vi "check if tag name exists.vi"(10 "name to locate":string, 11 "shared memory module configuration in":refnum<class "shared memory configuration.lvclass">) -> (0 "tag config":T1, 1 "index":i32, 2 "found?":bool, 3 "shared memory module configuration out":refnum<class "shared memory configuration.lvclass">)   [LabVIEW 2013, in "shared memory configuration.lvclass"]
doc: "***TODO***\n\n<B>Input Parameters</B>\n\n<B>name to locate</B> ***TODO***name to locate\n\n<B>shared memory module configuration in</B> ***TODO***shared memory module configuration in\n\n<B>Output Parameters</B>\n\n<B>tag config</B> ***TODO***tag config\n\n<B> * name</B> ***TODO***tag config.name\n\n<B> * data type</B> ***TODO***tag config.data type***enum values: Double,Single,I64,I32,I16,I8,U64,U32,U16,U8,Boolean,String,Array of Double,Array of Single,Array of I64,Array of I32,Array of I16,Array of I8,Array of U64,Array of U32,Array of U16,Array of U8,Array of Boolean,Array of String\n\n<B> * channel</B> ***TODO***tag config.channel\n\n<B>index</B> ***TODO***index\n\n<B>found?</B> ***TODO***found?\n\n<B>shared memory module configuration out</B> ***TODO***shared memory module configuration out"
uses:
  shared memory configuration.lvclass
  <vilib>/NI/Tag Bus Module Framework/channel/TBM channel.lvclass
  Line.ctl
  <vilib>/NI/Tag Bus/tag/Data Type.ctl
  <vilib>/NI/Tag Bus/tag/tag descriptor.lvclass
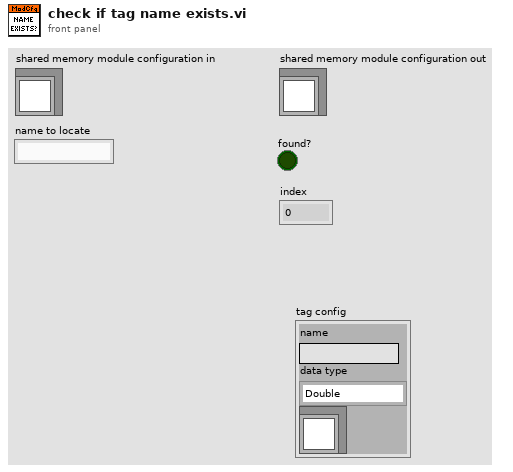
[diagram p1: front panel]
types:
  T1 = typedef "shared memory configuration.lvclass/Line.ctl" = cluster{"name":string, "data type":T2, "channel":refnum<class "TBM channel.lvclass">}
  T2 = typedef "tag bus.lvlib/tag descriptor.lvclass/Data Type.ctl" = enum16{"Double", "Single", "I64", "I32", "I16", "I8", "U64", "U32", "U16", "U8", "Boolean", "String", "Array of Double", "Array of Single", "Array of I64", "Array of I32", "Array of I16", "Array of I8", "Array of U64", "Array of U32", "Array of U16", "Array of U8", "Array of Boolean", "Array of String"}
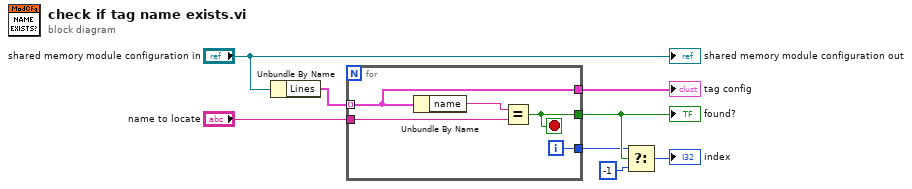
[diagram p0: block diagram]
diagram:
  n1 = Unbundle By Name("shared memory module configuration in") -> ("Lines"=w3:T1[])
  n2 = for {
    tunnel: w3 -> [w9] mode=indexing
    tunnel: "name to locate" -> [w12]
    tunnel: [w11] -> w6
    tunnel: [w10] -> w2
    tunnel: [w9] -> w4
    i -> [w10]
    stop <- w11 stop-if-true
    n3 = Unbundle By Name(w9) -> ("name"=w13:string)
    n4 = Equal?(x=w13, y=w12) -> (x = y?=w11:bool)
  }
  "found?" <- w6
  "tag config" <- w4
  n5 = Select(t=w2, s=w6, f=-1) -> (s? t:f=→"index":i32)
  "shared memory module configuration out" <- "shared memory module configuration in"
